vi "Copy All Shared Variables to Listbox.vi"(11 "Array":refnum<k21>[](array[refnum])) -> (2 "Listbox Data":string[][](array[string]))   [LabVIEW 2017, in "DTacq Plot Display Library.lvlib"]
uses:
  DTacq Plot Display Library.lvlib
  <resource>/objmgr/ni.var.rc
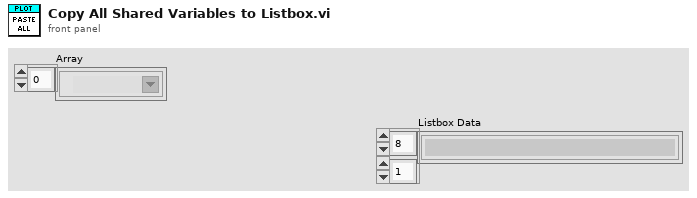
[diagram p1: front panel]
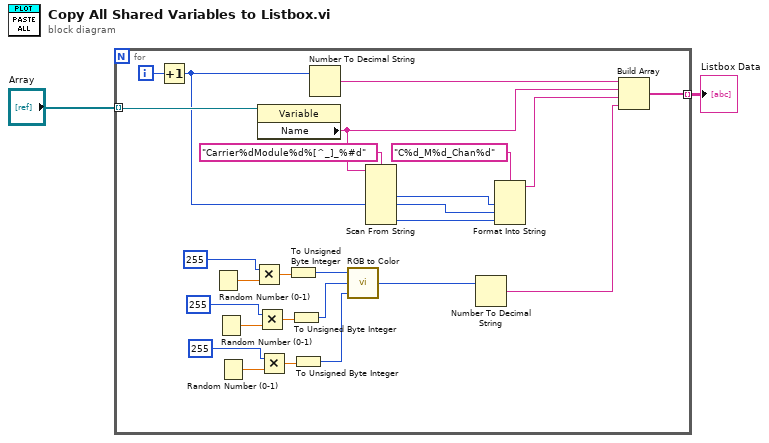
[diagram p0: block diagram]
diagram:
  n1 = for {
    tunnel: "Array" -> [w28] mode=indexing
    tunnel: [w21] -> w1 mode=indexing
    i -> [w7]
    n2 = Increment(x=w7) -> (x+1=w6:i32)
    n3 = Random Number (0-1)() -> (number: 0 to 1=w26:dbl)
    n4 = Random Number (0-1)() -> (number: 0 to 1=w19:dbl)
    n5 = Random Number (0-1)() -> (number: 0 to 1=w16:dbl)
    n6 = Multiply(x=255, y=w26) -> (x*y=w20:dbl)
    n7 = Multiply(x=255, y=w19) -> (x*y=w17:dbl)
    n8 = property class="Variable"(reference=w28) -> ("Name"=w23:string)  [unwired: 1 in, 2 out]
    n9 = Multiply(x=255, y=w16) -> (x*y=w14:dbl)
    n10 = To Unsigned Byte Integer(number=w20) -> (unsigned 8bit integer=w13:u8)
    n11 = To Unsigned Byte Integer(number=w17) -> (unsigned 8bit integer=w12:u8)
    n12 = To Unsigned Byte Integer(number=w14) -> (unsigned 8bit integer=w11:u8)
    n13 = Number To Decimal String(number=w6) -> (decimal integer string=w24:string)  [unwired: 1 in]
    n14 = call <vilib>:"RGB to Color.vi"("B"=w11, "G"=w12, "R"=w13) -> ("Color"=w10:u32)
    n15 = Scan From String(format string="Carrier%dModule%d%[^_]_%#d", input string=w23, default 2=w6) -> (output 1=w5:i32, output 2=w4:i32, output 4=w3:i32)  [unwired: 6 in, 3 out]
    n16 = Number To Decimal String(number=w10) -> (decimal integer string=w22:string)  [unwired: 1 in]
    n17 = Format Into String(format string="C%d_M%d_Chan%d", w5, w4, w3) -> (resulting string=w9:string)  [unwired: 2 in, 1 out]
    n18 = Build Array(w24, w23, w9, w22) -> (w21:string[])
  }
  "Listbox Data" <- w1
